vi "Driver Load.vi"(8 "error in (no error)":errorcluster, 10 "DriverID DriverType (\"\")":string) -> (0 "error out":errorcluster, 2 "Driver Component Path":path)   [LabVIEW 2011]
uses:
  client/client.lib/Spartan Client Version.vi
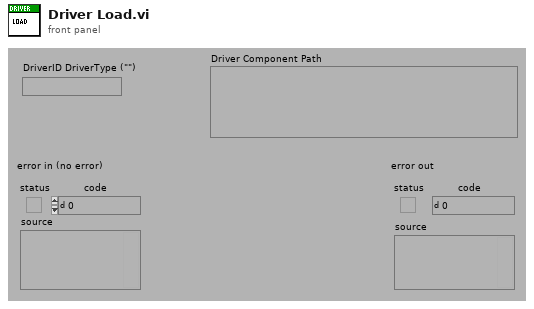
[diagram p1: front panel]
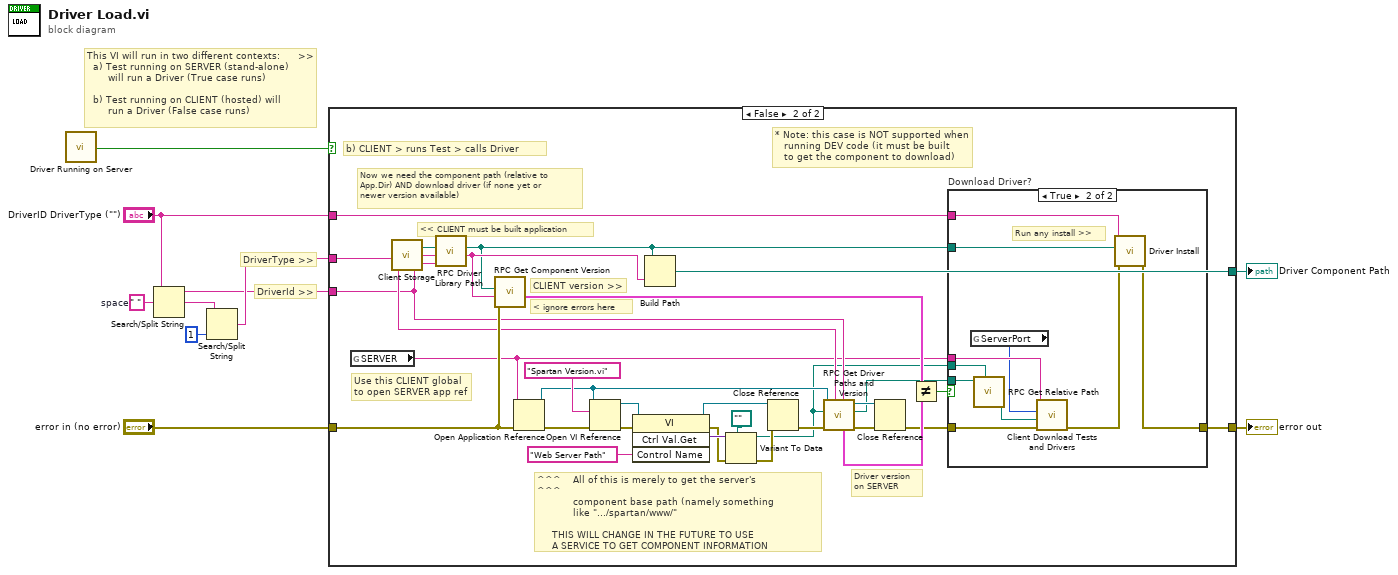
[diagram p0: block diagram]
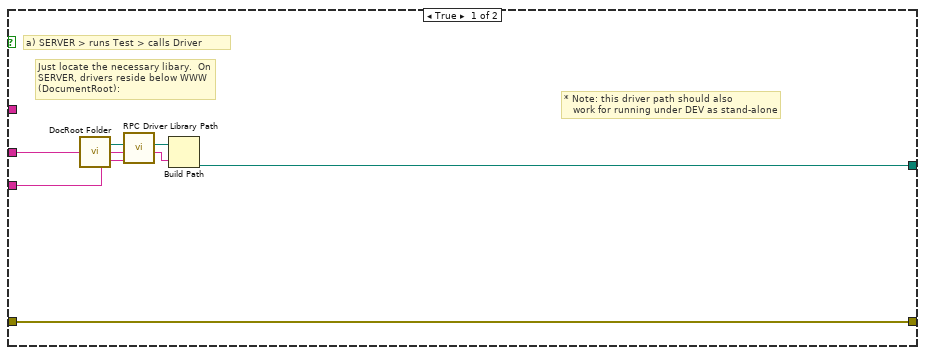
[diagram p2: hidden frame]
diagram:
  w10 = " "  # space
  # "This VI will run in two different contexts:      >>\n  a) Test running on SERVER (stand-alone)\n       will run a Driver (True case runs)\n\n  b) Test running on CLIENT (hosted) will\n       run a Driver (False case runs)"
  # "DriverId >>"
  # "DriverType >>"
  n1 = call "Driver Running on Server.vi"() -> ("Running on Server?"=w7:bool)
  n2 = Search/Split String(string="DriverID DriverType (\"\")", search string/char (-)=w10) -> (substring before match=w3:string, match + rest of string=w9:string)  [unwired: 2 out]
  n3 = Search/Split String(string=w9, offset (0)=1) -> (match + rest of string=w4:string)  [unwired: 3 out]
  n4 = case shown="False" w7 {
    tunnel: "error in (no error)" -> [w17 w47]
    tunnel: [w17 w26] -> w5
    tunnel: w4 -> [w15 w34]
    tunnel: w3 -> [w14 w33]
    tunnel: "DriverID DriverType (\"\")" -> [_ w21]
    tunnel: [w11 w19] -> w1
    frame True {
      # "* Note: this driver path should also\n   work for running under DEV as stand-alone"
      # "Just locate the necessary libary.  On\nSERVER, drivers reside below WWW\n(DocumentRoot):"
      # "a) SERVER > runs Test > calls Driver"
      n5 = call "DocRoot Folder.vi"() -> ("DocumentRoot Folder"=w16:path)  [unwired: 3 in]
      n6 = call "RPC Driver Library Path.vi"("Driver ID (\"\")"=w14, "Driver Type (\"\")"=w15, "Base Path (empty)"=w16) -> ("Driver Component Name"=w13:string, "Driver Library Path"=w12:path)  [unwired: 1 in, 6 out]
      n7 = Build Path(base path=w12, name or relative path=w13) -> (appended path=w11:path)
    }
    frame False {
      # "Driver version\non SERVER"
      # "^^^    All of this is merely to get the server's              ^^^\n            component base path (namely something\n            like \".../spartan/www/\"\n\n     THIS WILL CHANGE IN THE FUTURE TO USE\n     A SERVICE TO GET COMPONENT INFORMATION"
      # "Use this CLIENT global\nto open SERVER app ref"
      # "< ignore errors here"
      # "CLIENT version >>"
      # "* Note: this case is NOT supported when\n   running DEV code (it must be built\n   to get the component to download)"
      # "<< CLIENT must be built application"
      # "Now we need the component path (relative to\nApp.Dir) AND download driver (if none yet or\nnewer version available)"
      # "b) CLIENT > runs Test > calls Driver"
      n8 = global read "Spartan Client Version.vi" "SERVER"() -> (w25:string)
      n9 = call "Client Storage.vi"() -> ("Client Storage Path"=w18:path)  [unwired: 3 in]
      n10 = call "RPC Driver Library Path.vi"("Driver ID (\"\")"=w33, "Driver Type (\"\")"=w34, "Base Path (empty)"=w18) -> ("Driver Component Name"=w22:string, "Driver Library Path"=w20:path)  [unwired: 1 in, 6 out]
      n11 = call "RPC Get Component Version.vi"("error in (no error)"=w47, "Component (\"\")"=w22, "Component Library (empty)"=w20) -> ("Component Version"=w32:cluster{"Version":string, "Build Number":u32})  [unwired: 1 in, 7 out]
      n12 = Open Application Reference(8:w47, 11:w25) -> (0:w46:errorcluster, 3:w35:refnum<vi>)  [unwired: 2 out]
      n13 = Open VI Reference(application reference (local)=w35, vi path="Spartan Version.vi" ("y"), error in (no error)=w46) -> (vi reference=w42:refnum<vi>, error out=w43:errorcluster)  [unwired: 3 out]
      n14 = invoke class="VI" method="Ctrl Val.Get"(reference=w42, error in=w43, "Control Name"="Web Server Path" ("y")) -> (reference out=w37:refnum<vi>, error out=w40:errorcluster, "Get Control Value Variant"=w41:variant)  [unwired: 1 in, 1 out]
      n15 = Build Path(base path=w20, name or relative path=w22) -> (appended path=w19:path)
      n16 = Variant To Data(error in=w40, type=path "", Variant=w41) -> (data=w24:path, error out=w38:errorcluster)
      n17 = Close Reference(reference=w37, error in (no error)=w38) -> (error out=w36:errorcluster)
      n18 = call "RPC Get Driver Paths and Version.vi"("Driver ID (\"\")"=w33, "Driver Type (\"\")"=w34, "error in (no error)"=w36, "Base Path (empty)"=w24, "app reference (empty)"=w35) -> ("error out"=w29:errorcluster, "Driver Component Path"=w23:path, "app reference"=w27:refnum<vi>, "Component Version"=w31:cluster{"Version":string, "Build Number":u32})  [unwired: 1 in, 2 out]
      n19 = Close Reference(reference=w27, error in (no error)=w29) -> (error out=w28:errorcluster)
      n20 = Not Equal?(x=w32, y=w31) -> (x != y?=w30:bool)
      n21 = case "Download Driver?" shown="True" w30 {
        tunnel: w28 -> [w48 w58]
        tunnel: [w48 w52] -> w26
        tunnel: w25 -> [_ w57]
        tunnel: w24 -> [_ w56]
        tunnel: w23 -> [_ w55]
        tunnel: w20 -> [_ w54]
        tunnel: w21 -> [_ w51]
        frame False {
        }
        frame True {
          # "Run any install >>"
          n22 = global read "Spartan Client Version.vi" "ServerPort"() -> (w49:u16)
          n23 = call "RPC Get Relative Path.vi"("Base Path (empty)"=w56, "Absolute Path (empty)"=w55) -> ("Path Relative to Base"=w50:path)  [unwired: 3 out]
          n24 = call "Client Download Tests and Drivers.vi"("error in (no error)"=w58, "Test or Driver URL Path (empty)"=w50, "ServerPort (80)"=w49, "Server (\"\")"=w57) -> ("error out"=w53:errorcluster)  [unwired: 7 out]
          n25 = call "Driver Install.vi"("error in (no error)"=w53, "Driver Library Path"=w54, "DriverID DriverType (\"\")"=w51) -> ("error out"=w52:errorcluster)  [unwired: 1 in, 7 out]
        }
      }
    }
  }
  "error out" <- w5
  "Driver Component Path" <- w1
